vi "ListenAbort.vi"(0 "object in":refnum<class "Application.lvclass">, 5 "error in (no error)":errorcluster) -> (14 "object out":refnum<class "Application.lvclass">, 16 "Abort?":bool, 19 "error out":errorcluster)   [LabVIEW 2021, in "Application.lvclass"]
uses:
  Application.lvclass
  Application.lvclass/Application.ctl
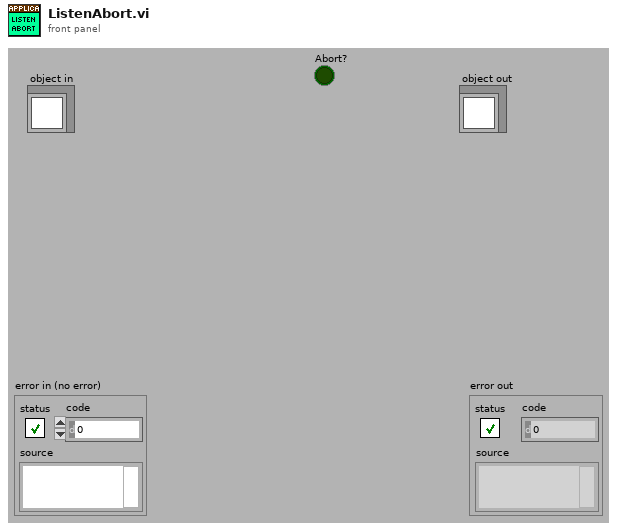
[diagram p1: front panel]
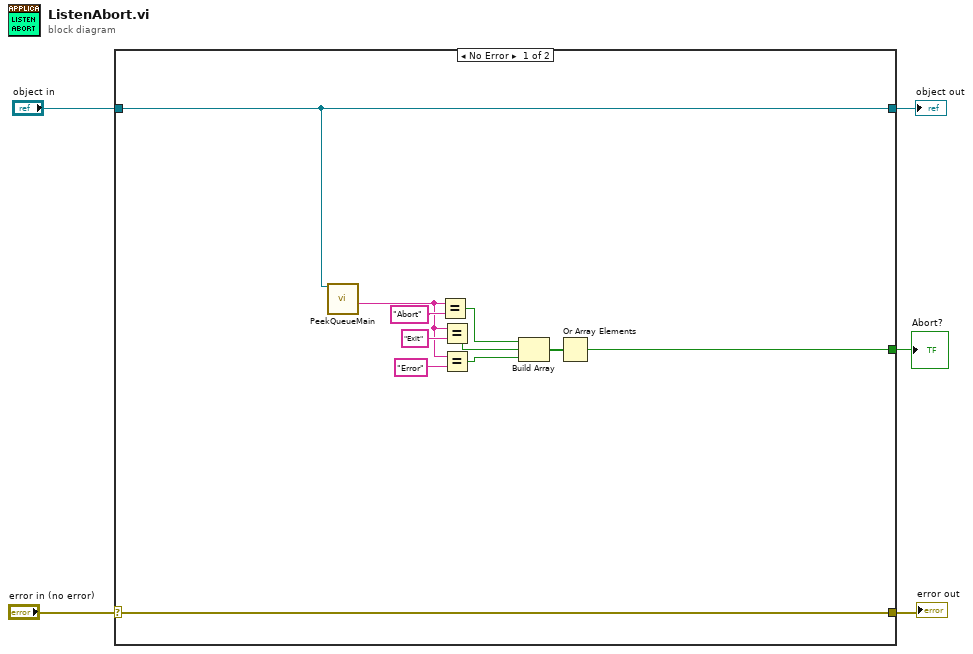
[diagram p0: block diagram]
diagram:
  n1 = case shown="No Error" "error in (no error)" {
    selector: "error in (no error)" -> [w16 w18]
    tunnel: [w16 w18] -> w4
    tunnel: [w7 w17] -> w2
    tunnel: "object in" -> [w7 w17]
    tunnel: [w6 _] -> w1
    frame No Error {
      n2 = call-dynamic "PeekQueueMain.vi"("object in"=w7) -> ("Message"=w8:string)  [unwired: 15 in, 3 out]
      n3 = Equal?(x=w8, y="Abort") -> (x = y?=w11:bool)
      n4 = Equal?(x=w8, y="Exit") -> (x = y?=w10:bool)
      n5 = Equal?(x=w8, y="Error") -> (x = y?=w12:bool)
      n6 = Build Array(w11, w10, w12) -> (w9:bool[])
      n7 = Or Array Elements(Boolean array=w9) -> (logical OR=w6:bool)
    }
    frame Error {
    }
  }
  "error out" <- w4
  "object out" <- w2
  "Abort?" <- w1
